vi "Receive.vi"(8 "error in (no error)":errorcluster, 10 "Transfer Group in":refnum<class "Transfer Group.lvclass">, 11 "UDP Transceiver in":refnum<class "DSF UDP Transceiver.lvclass">) -> (0 "error out":errorcluster, 2 "Transfer Group out":refnum<class "Transfer Group.lvclass">, 3 "UDP Transceiver out":refnum<class "DSF UDP Transceiver.lvclass">)   [LabVIEW 2017, in "DSF Core.lvlib" / "DSF UDP Transceiver.lvclass"]
uses:
  DSF UDP Transceiver.lvclass
  Classes/Transfer Group/Transfer Group.lvclass
  DSF UDP Transceiver.lvclass/DSF UDP Transceiver.ctl
  Read Datagram from Port.vi
  <vilib>/Utility/error.llb/Clear Errors.vi
  Classes/Transfer Group/Get Active Buffer.vi
  Classes/Buffer/Get Buffer Size.vi
  Throw Error.vi
  Throw Size Mismatch Error.vi
  Classes/Buffer/Write Buffer.vi
  Classes/Buffer/Write Buffer 1D U8.vi
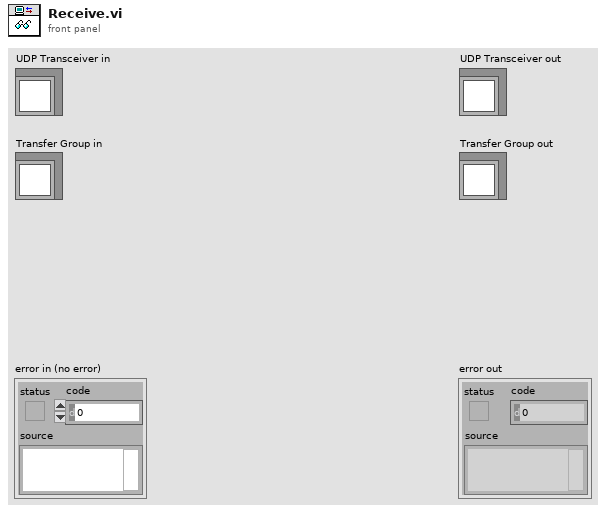
[diagram p1: front panel]
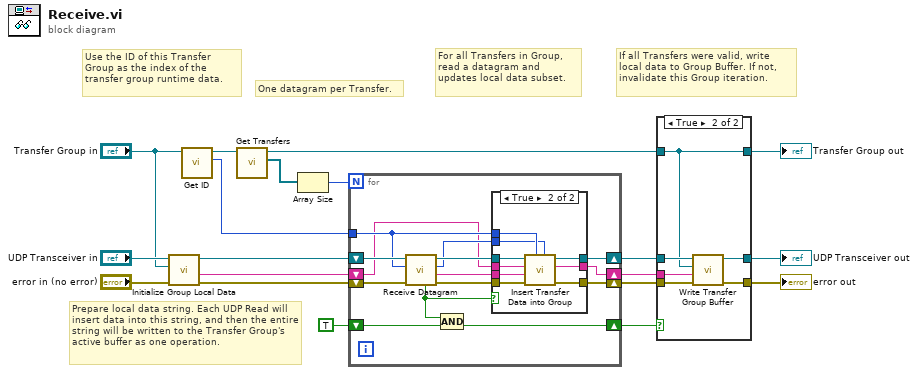
[diagram p0: block diagram]
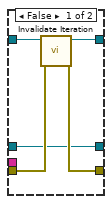
[diagram p3: hidden frame]
diagram:
  # "Prepare local data string. Each UDP Read will insert data into this string, and then the entire string will be written to the Transfer Group's active buffer as one operation."
  # "If all Transfers were valid, write local data to Group Buffer. If not, invalidate this Group iteration."
  # "Use the ID of this Transfer Group as the index of the transfer group runtime data."
  # "For all Transfers in Group, read a datagram and updates local data subset."
  # "One datagram per Transfer."
  n1 = call "Initialize Group Local Data.vi"("error in (no error)"="error in (no error)", "Transfer Group"="Transfer Group in", "UDP Transceiver in"="UDP Transceiver in") -> ("error out"=w6:errorcluster, "group data"=w5:string, "UDP Transceiver out"=w7:refnum<class "DSF UDP Transceiver.lvclass">)  [unwired: 6 in]
  n2 = call "Get ID.vi"("Transfer Group in"="Transfer Group in") -> ("id"=w16:i32, "Transfer Group out"=w19:refnum<class "Transfer Group.lvclass">)  [unwired: 9 in]
  n3 = call "Get Transfers.vi"("Transfer Group in"=w19) -> ("Transfers"=w17:refnum<class "Transfer.lvclass">[], "Transfer Group out"=w2:refnum<class "Transfer Group.lvclass">)  [unwired: 9 in]
  n4 = Array Size(array=w17) -> (size(s)=w18:i32)
  n5 = for {
    N: w18 -> [_]
    shift-right: [w27] -> w12
    shift-left: w6 -> [w32]
    shift-right: [w28] -> w14
    shift-left: w7 -> [w33]
    tunnel: w16 -> [w24]
    shift-right: [w25] -> w3
    shift-left: TRUE -> [w26]
    shift-right: [w21] -> w4
    shift-left: w5 -> [w22]
    n6 = call "Receive Datagram.vi"("error in (no error)"=w32, "transfer group id"=w24, "UDP Transceiver in"=w33) -> ("error out"=w30:errorcluster, "transfer data"=w29:string, "transfer id"=w23:i32, "UDP Transceiver out"=w31:refnum<class "DSF UDP Transceiver.lvclass">, "valid"=w20:bool)  [unwired: 4 in]
    n7 = Compound Arithmetic op=AND(w20, w26) -> (w25:bool)
    n8 = case shown="True" w20 {
      tunnel: w31 -> [w36 w45]
      tunnel: w30 -> [w35 w44]
      tunnel: w29 -> [_ w42]
      tunnel: [w36 w37] -> w28
      tunnel: [w35 w43] -> w27
      tunnel: w24 -> [_ w41]
      tunnel: w23 -> [_ w40]
      tunnel: w22 -> [w34 w38]
      tunnel: [w34 w39] -> w21
      frame False {
      }
      frame True {
        n9 = call "Insert Transfer Data into Group.vi"("transfer id"=w40, "transfer group id"=w41, "error in (no error)"=w44, "transfer data"=w42, "group data in"=w38, "UDP Transceiver in"=w45) -> ("error out"=w43:errorcluster, "group data out"=w39:string, "UDP Transceiver out"=w37:refnum<class "DSF UDP Transceiver.lvclass">)  [unwired: 3 in]
      }
    }
  }
  n10 = case shown="True" w3 {
    tunnel: w14 -> [w46 w56]
    tunnel: [w46 w55] -> w13
    tunnel: w12 -> [w50 w54]
    tunnel: [w49 w53] -> w11
    tunnel: w4 -> [_ w52]
    tunnel: w2 -> [w48 w51]
    tunnel: [w47 w51] -> w1
    frame False {
      n11 = call "Invalidate Iteration.vi"("error in (no error)"=w50, "Transfer Group in"=w48) -> ("error out"=w49:errorcluster, "Transfer Group out"=w47:refnum<class "Transfer Group.lvclass">)  [unwired: 8 in]
    }
    frame True {
      n12 = call "Write Transfer Group Buffer.vi"("error in (no error)"=w54, "data"=w52, "Transfer Group"=w51, "UDP Transceiver in"=w56) -> ("error out"=w53:errorcluster, "UDP Transceiver out"=w55:refnum<class "DSF UDP Transceiver.lvclass">)  [unwired: 6 in]
    }
  }
  "error out" <- w11
  "UDP Transceiver out" <- w13
  "Transfer Group out" <- w1
